vi "RPC Register.vi"(8 "error in (no error)":errorcluster, 11 "OOP Server in":refnum<class "OOP Server.lvclass">) -> (0 "error out":errorcluster, 3 "OOP Server out":refnum<class "OOP Server.lvclass">)   [LabVIEW 2019, in "OOP Server.lvclass"]
uses:
  OOP Server.lvclass
  OOP Server.lvclass/OOP Server.ctl
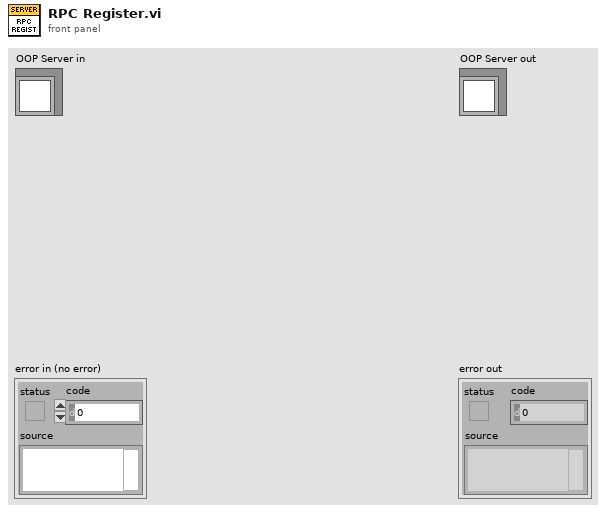
[diagram p1: front panel]
types:
  T1 = typedef "OOP Server.lvclass/Server Internal UEs.ctl" = cluster{"Invoke Internal UE":refnum<user-event>, "Query Internal UE":refnum<user-event>, "Register Internal UE":refnum<user-event>}
  T2 = typedef "OOP Server.lvclass/Server gRPC UEs.ctl" = cluster{"Invoke gRPC UEs":T3, "Query gRPC UEs":T3, "Register gRPC UEs":T3}
  T3 = typedef "gprc-lvsupport.lvlib/gRPCId Cluster UE.ctl" = refnum<user-event>
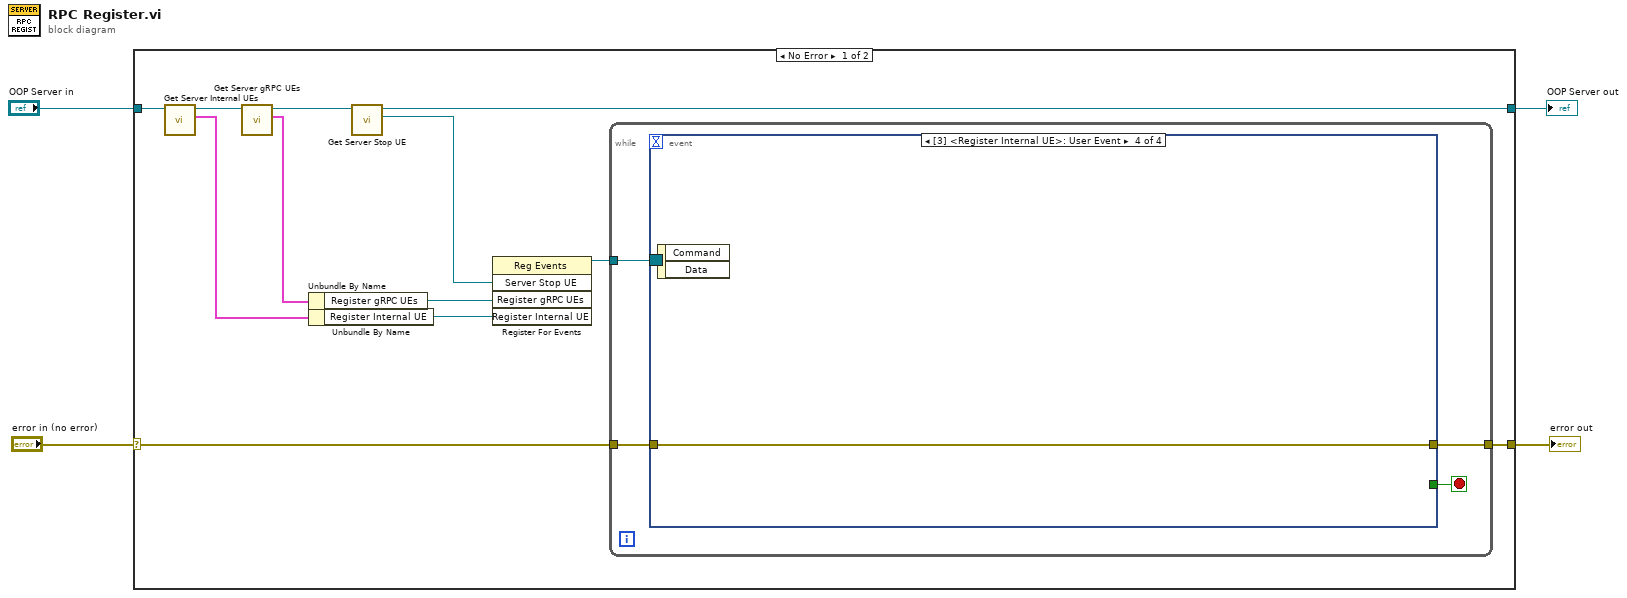
[diagram p0: block diagram]
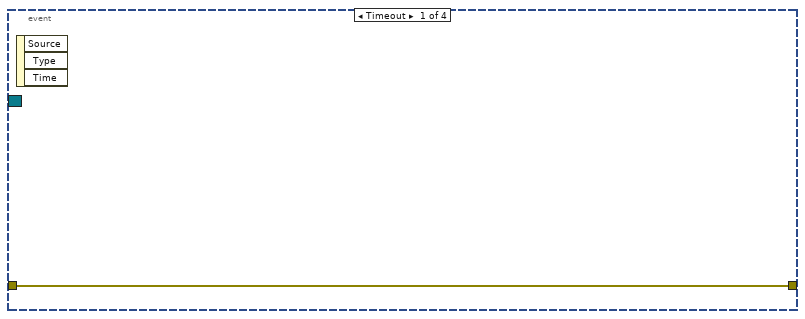
[diagram p2: hidden frame]
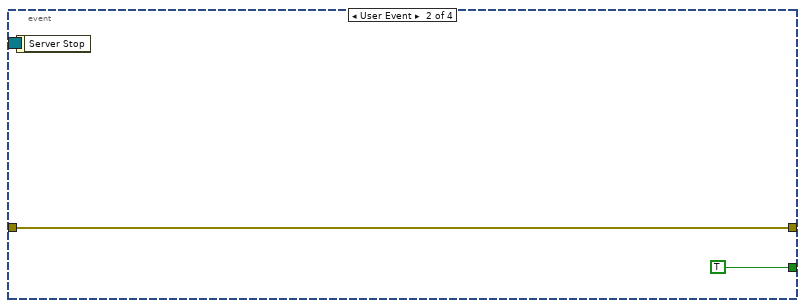
[diagram p3: hidden frame]
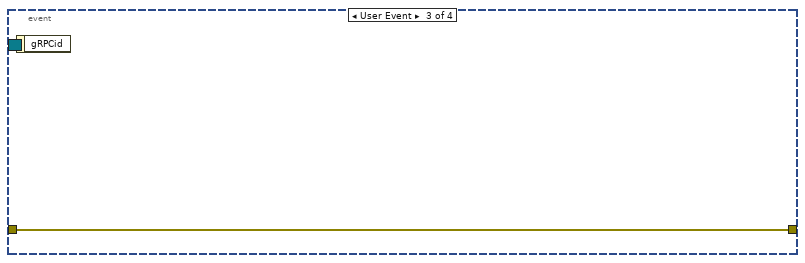
[diagram p4: hidden frame]
diagram:
  n1 = case shown="No Error" "error in (no error)" {
    selector: "error in (no error)" -> [w6 w27]
    tunnel: [w5 w27] -> w3
    tunnel: [w14 w26] -> w1
    tunnel: "OOP Server in" -> [w10 w26]
    frame No Error {
      n2 = call "Get Server Internal UEs.vi"("OOP Server in"=w10) -> ("Server Internal UEs"=w8:T1, "OOP Server out"=w9:refnum<class "OOP Server.lvclass">)  [unwired: 9 in]
      n3 = call "Get Server gRPC UEs.vi"("OOP Server in"=w9) -> ("Server gRPC UEs"=w12:T2, "OOP Server out"=w16:refnum<class "OOP Server.lvclass">)  [unwired: 9 in]
      n4 = Unbundle By Name(w12) -> ("Register gRPC UEs"=w11:T3)
      n5 = Unbundle By Name(w8) -> ("Register Internal UE"=w7:refnum<user-event>)
      n6 = call "Get Server Stop UE.vi"("OOP Server in"=w16) -> ("Server Stop UE"=w15:refnum<user-event>, "OOP Server out"=w14:refnum<class "OOP Server.lvclass">)  [unwired: 9 in]
      n7 = register-events(w15, w11, w7) -> (reference out=w13:refnum<event-registration>)  [unwired: 2 in, 1 out]
      n8 = while {
        tunnel: w13 -> [w20]
        tunnel: w6 -> [w18]
        tunnel: [w17] -> w5
        stop <- w19 stop-if-true
        n9 = event shown="[3] <Register Internal UE>: User Event" {
          selector: w20 -> [_ _ _ _]
          dyn-events: _ -> [_ _ _ _]
          timeout: _ -> [_ _ _ _]
          tunnel: [_ TRUE _ _] -> w19
          tunnel: w18 -> [w21 w22 w24 w25]
          tunnel: [w21 w22 w24 w25] -> w17
          event Timeout {
            n10 = event-data() -> ()  [unwired: 1 in, 3 out]
          }
          event User Event {
            n11 = event-data() -> ()  [unwired: 1 in, 1 out]
          }
          event User Event {
            n12 = event-data() -> ()  [unwired: 1 in, 1 out]
          }
          event User Event {
            n13 = event-data() -> ()  [unwired: 1 in, 2 out]
          }
        }
      }
    }
    frame Error {
    }
  }
  "error out" <- w3
  "OOP Server out" <- w1
